vi "Printing media.vi"(8 "error in (no error)":errorcluster, 10 "send on  barcode printer":string, 11 "printer name":string="TSC TA3123") -> (0 "error out":errorcluster)   [LabVIEW 2015]
uses:
  <vilib>/Utility/NIReport.llb/Append Report Text (str wrap).vi
  <vilib>/Utility/NIReport.llb/NI_report.lvclass
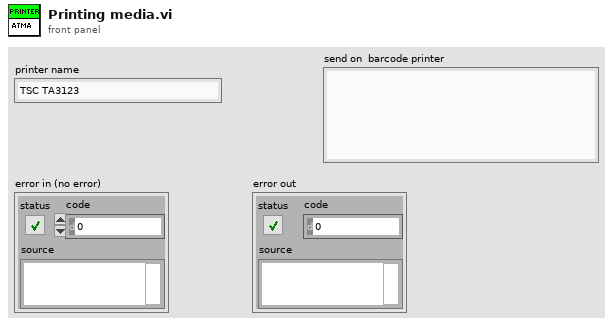
[diagram p1: front panel]
types:
  T1 = enum16{"Standard Report", "HTML", "Word", "Excel"}
  T2 = enum16{"maximized", "minimized", "normal", "no change"}
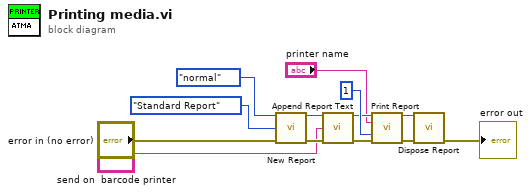
[diagram p0: block diagram]
diagram:
  n1 = call <vilib>:"New Report.vi"("window state (normal)"=T2."normal", "report type"=T1."Standard Report", "error in (no error)"="error in (no error)") -> ("report out"=w11:refnum<class "NI_report.lvclass">, "error out"=w12:errorcluster)  [unwired: 11 in]
  n2 = call-poly <vilib>:"Append Report Text.vi"("report in"=w11, "text"="send on  barcode printer", "error in (no error)"=w12) -> ("report out"=w9:refnum<class "NI_report.lvclass">, "error out"=w10:errorcluster)  [unwired: 9 in, 2 out]
  n3 = call-dynamic "Print Report.vi"("report in"=w9, "printer name (default)"="printer name", "number of copies (1)"=1, "error in (no error)"=w10) -> ("report out"=w7:refnum<class "NI_report.lvclass">, "error out"=w8:errorcluster)  [unwired: 10 in]
  n4 = call-dynamic "Dispose Report.vi"("report in"=w7, "error in (no error)"=w8) -> ("error out"=→"error out":errorcluster)  [unwired: 13 in]
